vi "Write JSON reader.lvclass.vi"(8 "error in (no error)":errorcluster, 10 "JSON reader.lvclass":refnum<class "JSON reader.lvclass">, 11 "File interpreter in":refnum<class "File interpreter.lvclass">) -> (0 "error out":errorcluster, 3 "File interpreter out":refnum<class "File interpreter.lvclass">)   [LabVIEW 2018, in "File interpreter.lvclass"]
uses:
  File interpreter.lvclass
  JSON reader/JSON reader.lvclass
  File interpreter.lvclass/File interpreter.ctl
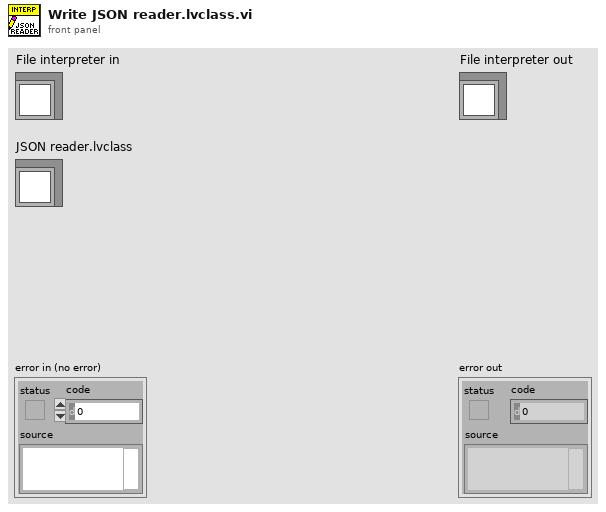
[diagram p1: front panel]
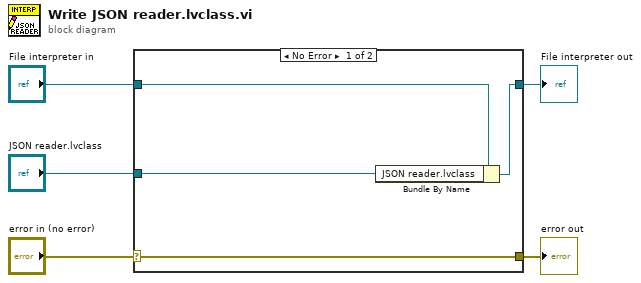
[diagram p0: block diagram]
diagram:
  n1 = case shown="No Error" "error in (no error)" {
    selector: "error in (no error)" -> [w9 w10]
    tunnel: [w9 w10] -> w4
    tunnel: [w7 w11] -> w2
    tunnel: "File interpreter in" -> [w8 w11]
    tunnel: "JSON reader.lvclass" -> [w6 _]
    frame No Error {
      n2 = Bundle By Name(cluster=w8, "JSON reader.lvclass"=w6) -> (w7:refnum<class "File interpreter.lvclass">)
    }
    frame Error {
    }
  }
  "error out" <- w4
  "File interpreter out" <- w2
